vi "Get Manager QueryAllChannels Request.vi"(8 "error in (no error)":errorcluster, 11 "gRPCid":T1) -> (0 "error out":errorcluster, 2 "Message Data":T2, 3 "gRPCid out":T1)   [LabVIEW 2021, in "CIF_Manager_server.lvlib" / "Manager.lvclass"]
uses:
  Manager.lvclass
  <vilib>/gRPC/LabVIEW gRPC Library/Shared/grpcId.ctl
  <vilib>/gRPC/gRPC Server and Client Template [2]/Server Template/RPC Messages/Get package_templatemessage.vi/c750bf2f-d32b-4a25-a00a-5db67bc240fd.vi
  <vilib>/gRPC/gRPC Server and Client Template [2]/Server Template/RPC Messages/Get package_templatemessage.vi/2ed25e12-861d-4677-8ead-ace2906b2041.vi
  <vilib>/gRPC/LabVIEW gRPC Library/Shared/TranslateGrpcError.vi
  <vilib>/gRPC/LabVIEW gRPC Library/Server API/Server/Get Server DLL Path.vi
  <vilib>/Utility/error.llb/Error Cluster From Error Code.vi
  Manager.lvclass/Manager.ctl
  CIF_Manager_server.lvlib
  <vilib>/gRPC/LabVIEW gRPC Library/grpc-lvsupport-release.lvlib
  RPC Messages/cif_channelcore_ChannelDirection.ctl
  RPC Messages/cif_channelcore_ChannelFilter.ctl
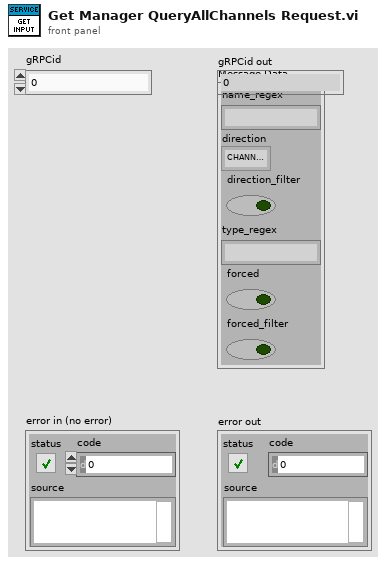
[diagram p1: front panel]
types:
  T1 = typedef "grpc-lvsupport-release.lvlib/grpcId.ctl" = u64
  T2 = typedef "CIF_Manager_server.lvlib/cif_channelcore_ChannelFilter.ctl" = cluster{"name_regex":string, "direction":T3, "direction_filter":bool, "type_regex":string, "forced":bool, "forced_filter":bool}
  T3 = typedef "CIF_Manager_server.lvlib/cif_channelcore_ChannelDirection.ctl" = enum32{"CHANNELDIRECTION_UNKNOWN", "CHANNELDIRECTION_PUBLISHER", "CHANNELDIRECTION_SUBSCRIBER"}
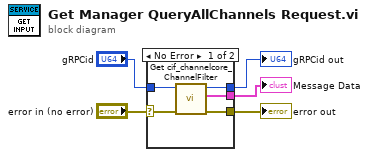
[diagram p0: block diagram]
diagram:
  n1 = case shown="No Error" "error in (no error)" {
    selector: "error in (no error)" -> [w10 w12]
    tunnel: [w9 w12] -> w4
    tunnel: [w8 _] -> w3
    tunnel: "gRPCid" -> [w7 w11]
    tunnel: [w6 w11] -> w1
    frame No Error {
      n2 = call "Get cif_channelcore_ChannelFilter.vi"("error in (no error)"=w10, "gRPCid"=w7) -> ("error out"=w9:errorcluster, "package_templatemessage"=w8:T2, "gRPCid out"=w6:T1)  [unwired: 7 in]
    }
    frame Error {
    }
  }
  "error out" <- w4
  "Message Data" <- w3
  "gRPCid out" <- w1
